vi "FlatToRichcif_management_common_ChannelFilter.vi"(5 "OutputClusterType":T1, 11 "InputCluster":T3) -> (3 "OutputCluster":T1)   [LabVIEW 2021, in "CIF_Manager_client.lvlib"]
uses:
  CIF_Manager_client.lvlib
  cif_management_common_ChannelFilter_Flat.ctl
  cif_management_common_ChannelDirection.ctl
  cif_management_common_ChannelFilter.ctl
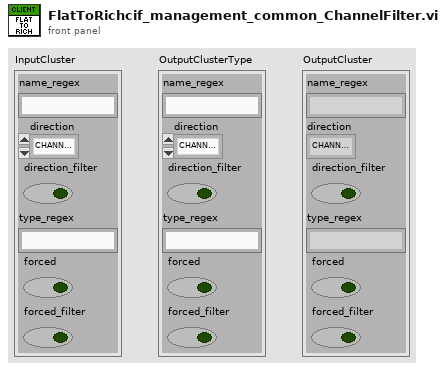
[diagram p1: front panel]
types:
  T1 = typedef "CIF_Manager_client.lvlib/cif_management_common_ChannelFilter.ctl" = cluster{"name_regex":string, "direction":T2, "direction_filter":bool, "type_regex":string, "forced":bool, "forced_filter":bool}
  T2 = typedef "CIF_Manager_client.lvlib/cif_management_common_ChannelDirection.ctl" = enum32{"CHANNELDIRECTION_UNKNOWN", "CHANNELDIRECTION_PUBLISHER", "CHANNELDIRECTION_SUBSCRIBER"}
  T3 = typedef "CIF_Manager_client.lvlib/cif_management_common_ChannelFilter_Flat.ctl" = cluster{"name_regex":string, "direction":T2, "direction_filter":bool, "type_regex":string, "forced":bool, "forced_filter":bool}
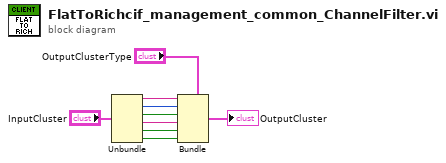
[diagram p0: block diagram]
diagram:
  n1 = Unbundle "Unbundle"("InputCluster") -> ("name_regex"=w6:string, "direction"=w5:T2, "direction_filter"=w4:bool, "type_regex"=w3:string, "forced"=w2:bool, "forced_filter"=w1:bool)
  n2 = Bundle "Bundle"(cluster="OutputClusterType", "name_regex"=w6, "direction"=w5, "direction_filter"=w4, "type_regex"=w3, "forced"=w2, "forced_filter"=w1) -> (→"OutputCluster":T1)
